vi "Reduced_Density_Matrix.vi"(8 "error in (no error)":errorcluster, 10 "Qubits to Keep":i32[](array[numeric])=[0, 2, 1], 11 "QuWire in":refnum<class "QuWire.lvclass">) -> (0 "error out":errorcluster, 1 "Indices":i32[](array[numeric]), 2 "Reduced Density Matrix":cdb[][](array[numeric]), 3 "QuWire out":refnum<class "QuWire.lvclass">)   [LabVIEW 2020, in "QuWire.lvclass"]
uses:
  QuWire.lvclass
  QuWire.lvclass/QuWire.ctl
  a1189c4a-9114-4079-95c2-ba167920f6d7.vi
  SimAlg/PrllPerElement/PrllPerElmnt.lvclass
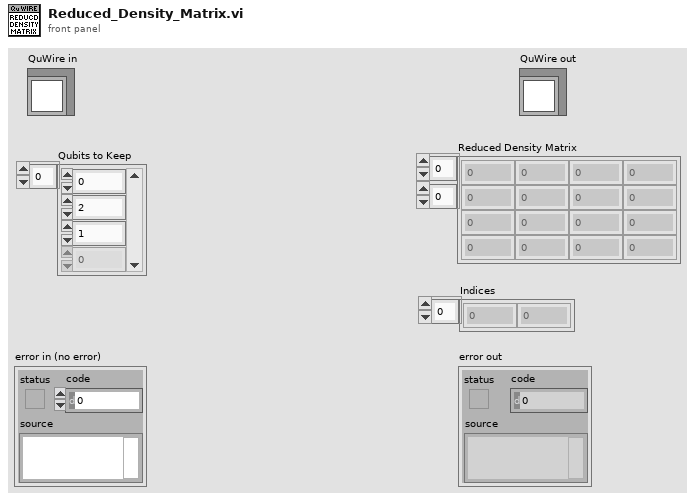
[diagram p1: front panel]
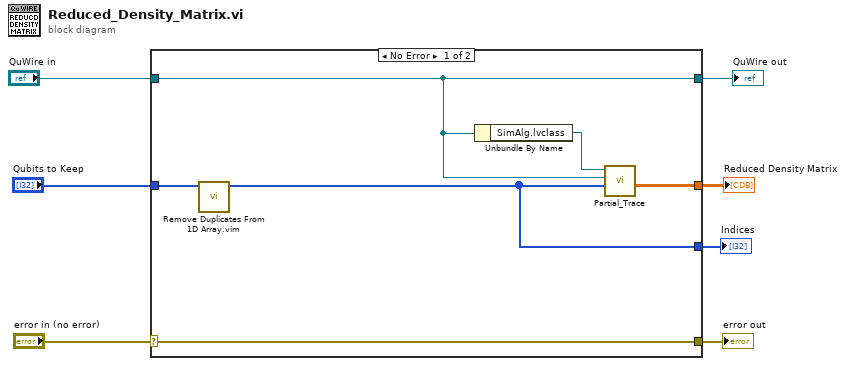
[diagram p0: block diagram]
diagram:
  n1 = case shown="No Error" "error in (no error)" {
    selector: "error in (no error)" -> [w13 w15]
    tunnel: [w13 w15] -> w6
    tunnel: [w11 _] -> w5
    tunnel: "QuWire in" -> [w10 w14]
    tunnel: [w10 w14] -> w3
    tunnel: "Qubits to Keep" -> [w9 _]
    tunnel: [w8 _] -> w1
    frame No Error {
      n2 = call "Remove Duplicates From 1D Array.vim"("array"=w9) -> ("array with duplicates removed"=w8:i32[])  [unwired: 10 in]
      n3 = Unbundle By Name(w10) -> ("SimAlg.lvclass"=w12:refnum<class "PrllPerElmnt.lvclass">)
      n4 = call-dynamic "Partial_Trace.vi"("Qubits to Keep"=w8, "QuWire in"=w10, "SimAlg in"=w12) -> ("Reduced Density Matrix"=w11:cdb[][])  [unwired: 5 in, 3 out]
    }
    frame Error {
    }
  }
  "error out" <- w6
  "Reduced Density Matrix" <- w5
  "QuWire out" <- w3
  "Indices" <- w1
